vi "addLineToProjections.vi"(9 "current volume":T3, 10 "line":T2, 11 "buffers":T1) -> (3 "buffers out":T1)   [LabVIEW 2010]
uses:
  volume_info.ctl
  line_info.ctl
  projection buffers.ctl
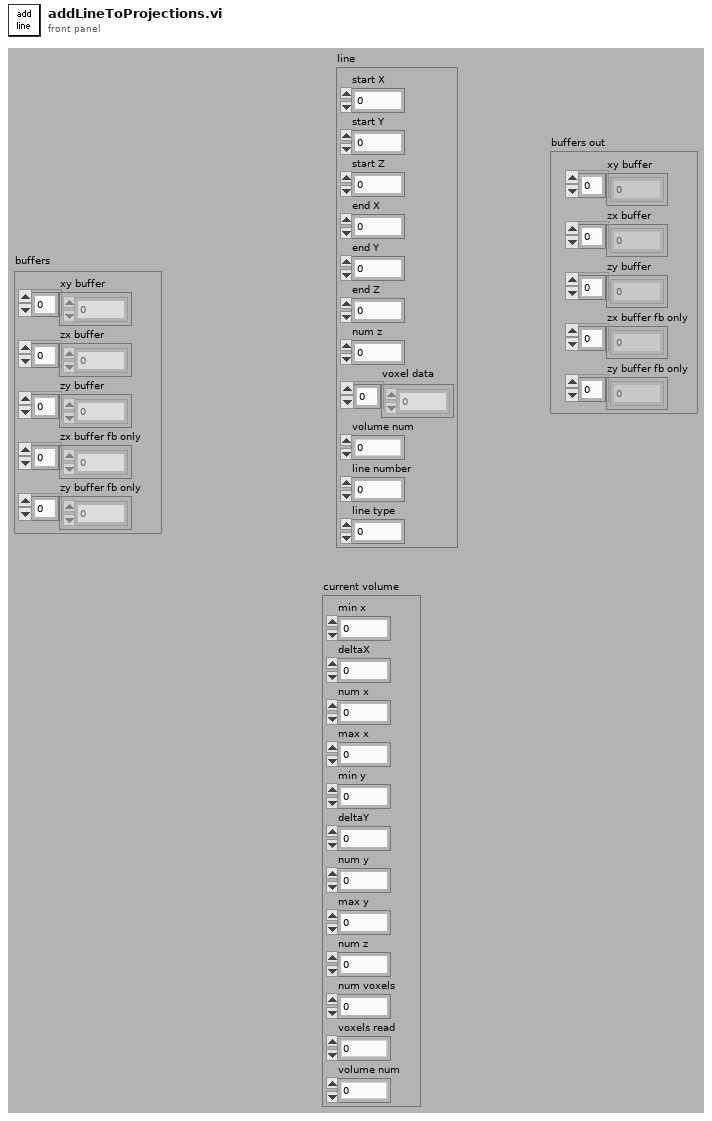
[diagram p1: front panel]
types:
  T1 = typedef "projection buffers.ctl" = cluster{"xy buffer":u32[], "zx buffer":u32[], "zy buffer":u32[], "zx buffer fb only":u32[], "zy buffer fb only":u32[]}
  T2 = typedef "line_info.ctl" = cluster{"start X":i16, "start Y":i16, "start Z":i16, "end X":i16, "end Y":i16, "end Z":i16, "num z":u8, "voxel data":u32[], "volume num":u32, "line number":u16, "line type":u16}
  T3 = typedef "volume_info.ctl" = cluster{"min x":i16, "deltaX":dbl, "num x":u32, "max x":i16, "min y":i16, "deltaY":dbl, "num y":u32, "max y":i16, "num z":u32, "num voxels":u32, "voxels read":u32, "volume num":u32}
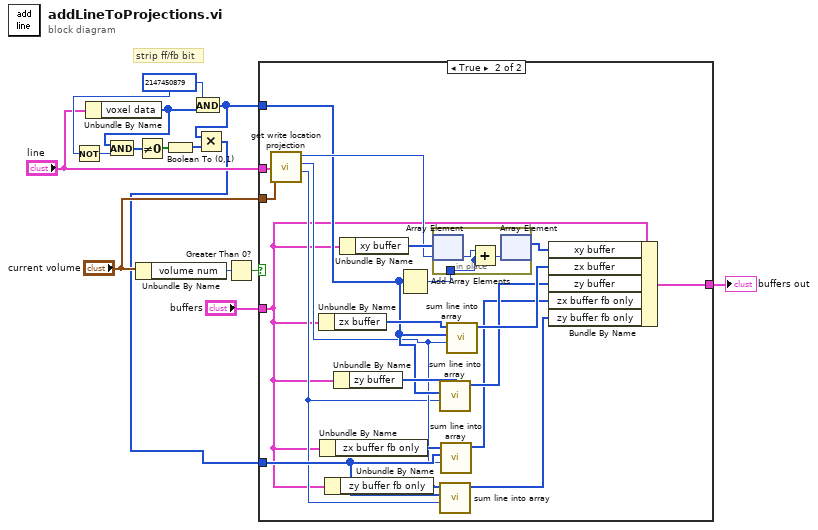
[diagram p0: block diagram]
diagram:
  w6 = u32 2147450879
  # "strip ff/fb bit"
  n1 = Not(x=w6) -> (.not. x?=w5:u32)
  n2 = Unbundle By Name("line") -> ("voxel data"=w10:u32[])
  n3 = And(x=w10, y=w5) -> (x .and. y?=w7:u32[])
  n4 = Unbundle By Name("current volume") -> ("volume num"=w13:u32)
  n5 = Not Equal To 0?(x=w7) -> (x != 0?=w8:bool[])
  n6 = Boolean To (0,1)(Boolean=w8) -> (0, 1=w9:i16[])
  n7 = And(x=w6, y=w10) -> (x .and. y?=w3:u32[])
  n8 = Multiply(x=w3, y=w9) -> (x*y=w2:u32[])
  n9 = Greater Than 0?(x=w13) -> (x > 0?=w12:bool)
  n10 = case shown="True" w12 {
    tunnel: "current volume" -> [_ w35]
    tunnel: "buffers" -> [w15 w22]
    tunnel: "line" -> [_ w31]
    tunnel: w3 -> [_ w28]
    tunnel: w2 -> [_ w25]
    tunnel: [w15 w16] -> w1
    frame False {
    }
    frame True {
      n11 = call "get write location projection.vi"("current volume"=w35, "line"=w31) -> ("zy insert point"=w23:u32, "zx insert point"=w24:u32, "xy insert point"=w33:u32)  [unwired: 7 in]
      n12 = Unbundle By Name(w22) -> ("zx buffer"=w30:u32[])
      n13 = Unbundle By Name(w22) -> ("zx buffer fb only"=w26:u32[])
      n14 = Unbundle By Name(w22) -> ("zy buffer fb only"=w27:u32[])
      n15 = Unbundle By Name(w22) -> ("zy buffer"=w29:u32[])
      n16 = Unbundle By Name(w22) -> ("xy buffer"=w34:u32[])
      n17 = Add Array Elements(numeric array=w28) -> (sum=w32:u32)
      n18 = in-place {
        in-place-border: w32 -> [w36]
        n19 = in-place-array #1(w34, w33) -> (w37:u32)
        n20 = Add(x=w37, y=w36) -> ()  [unwired: 1 out]
        n21 = in-place-array #1(w36) -> (w21:u32[])  [unwired: 1 out]
      }
      n22 = call "sum line into array.vi"("insert location"=w23, "array to sum in"=w28, "array"=w29) -> ("array out"=w19:u32[])  [unwired: 8 in]
      n23 = call "sum line into array.vi"("insert location"=w23, "array to sum in"=w25, "array"=w27) -> ("array out"=w17:u32[])  [unwired: 8 in]
      n24 = call "sum line into array.vi"("insert location"=w24, "array to sum in"=w25, "array"=w26) -> ("array out"=w18:u32[])  [unwired: 8 in]
      n25 = call "sum line into array.vi"("insert location"=w24, "array to sum in"=w28, "array"=w30) -> ("array out"=w20:u32[])  [unwired: 8 in]
      n26 = Bundle By Name(cluster=w22, "xy buffer"=w21, "zx buffer"=w20, "zy buffer"=w19, "zx buffer fb only"=w18, "zy buffer fb only"=w17) -> (w16:T1)
    }
  }
  "buffers out" <- w1
